vi "Get Vector Components.vi"(8 "error in":errorcluster, 11 "PVector in":refnum<class "PVector.lvclass">) -> (0 "error out":errorcluster, 1 "Y":dbl, 2 "X":dbl, 3 "PVector out":refnum<class "PVector.lvclass">)   [LabVIEW 2016, in "PVector.lvclass"]
doc: "Return vector V individual components Vx and Vy"
uses:
  PVector.lvclass
  PVector.lvclass/PVector.ctl
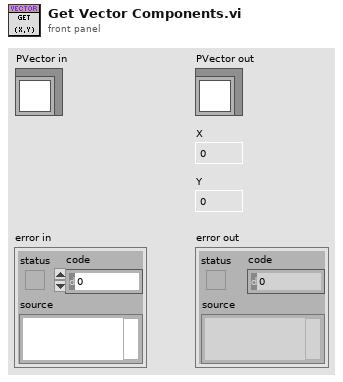
[diagram p1: front panel]
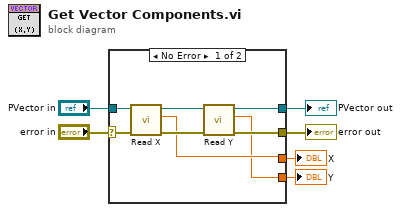
[diagram p0: block diagram]
diagram:
  n1 = case shown="No Error" "error in" {
    selector: "error in" -> [w11 w16]
    tunnel: [w9 w16] -> w5
    tunnel: [w10 w15] -> w3
    tunnel: "PVector in" -> [w14 w15]
    tunnel: [w8 _] -> w2
    tunnel: [w7 _] -> w1
    frame No Error {
      n2 = call "Read X.vi"("error in"=w11, "PVector in"=w14) -> ("error out"=w12:errorcluster, "X"=w8:dbl, "PVector out"=w13:refnum<class "PVector.lvclass">)  [unwired: 7 in]
      n3 = call "Read Y.vi"("error in"=w12, "PVector in"=w13) -> ("error out"=w9:errorcluster, "Y"=w7:dbl, "PVector out"=w10:refnum<class "PVector.lvclass">)  [unwired: 7 in]
    }
    frame Error {
    }
  }
  "error out" <- w5
  "PVector out" <- w3
  "X" <- w2
  "Y" <- w1
